vi "AddCORS.vi"(8 "error in (no error)":errorcluster, 11 "Web Request in":refnum<class "Web Request.lvclass">) -> (0 "error out":errorcluster, 3 "Web Request out":refnum<class "Web Request.lvclass">)   [LabVIEW 2017]
doc: "This VI adds the necessary headers to allow requests that use CORS. This is needed to send HTTP-Requests from a different Webserver to this Webserver. E.g. requesting the Data from a NXG-WebVI."
uses:
  <vilib>/wsapi/Web Request.lvclass
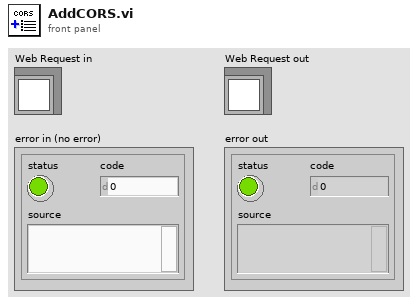
[diagram p1: front panel]
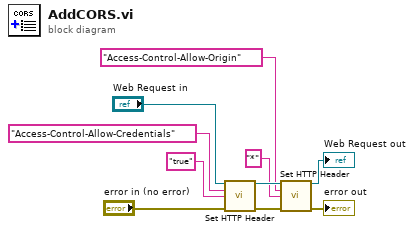
[diagram p0: block diagram]
diagram:
  n1 = call <vilib>:"Set HTTP Header.vi"("LabVIEW Web Service Request"="Web Request in", "header"="Access-Control-Allow-Credentials", "header value"="true", "error in (no error)"="error in (no error)") -> ("LabVIEW Web Service Request out"=w3:refnum<class "Web Request.lvclass">, "error out"=w8:errorcluster)  [unwired: 10 in]
  n2 = call <vilib>:"Set HTTP Header.vi"("LabVIEW Web Service Request"=w3, "header"="Access-Control-Allow-Origin", "header value"="*", "error in (no error)"=w8) -> ("LabVIEW Web Service Request out"=→"Web Request out":refnum<class "Web Request.lvclass">, "error out"=→"error out":errorcluster)  [unwired: 10 in]
